vi "discrete_controller.run.vi"(4 "reset? (F)":bool, 5 "error_offset (0)":dbl format="%#_13g", 6 "outut limits (100/0)":cluster{"max_limit":dbl, "min_limit":dbl}={"max_limit"=100.0, "min_limit"=0.0}, 7 "discrete_coefficients":cluster{"b0...bn":dbl[], "a1...an":dbl[]}={"b0...bn"=[0.0, 0.0, 0.0, 0.0], "a1...an"=[0.0, 0.0, 0.0, 0.0]}, 9 "initial_output (0)":dbl format="%#_13g", 10 "feedback":dbl format="%#_13g", 11 "setpoint":dbl format="%#_13g") -> (3 "controller_output":dbl)   [LabVIEW 2015, in "discrete_control_systems.lvlib"]
doc: "This VI implements a SISO discrete controller configured according to the provided discrete coefficients for a difference equation of the form:\n\ny(k) = b0*x(k) + b1*x(k-1) + b2*x(k-2) + bn*x(k-n) - ( a1*y(k-1) + a2*y(k-2) + a3*y(k-3) + an*y(k-n) )\n\nThe output will be coerced withing Min Limit and Max Limit. After resetting the controller, the output will be initialized to the initial output selected. This helps implement bumpless transfers between open loop and closed loop operations."
uses:
  discrete_control_systems.lvlib
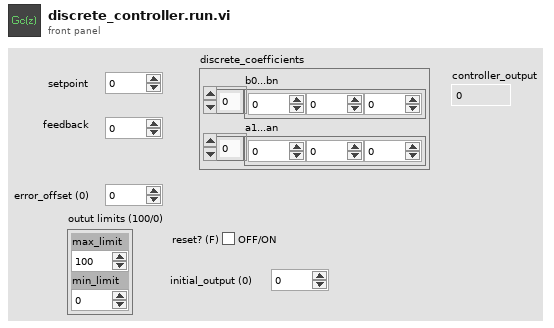
[diagram p1: front panel]
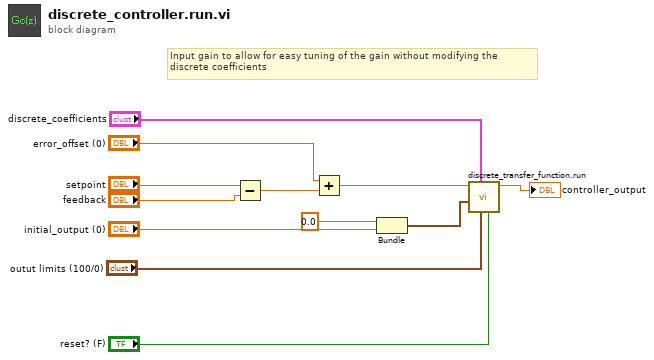
[diagram p0: block diagram]
diagram:
  # "Input gain to allow for easy tuning of the gain without modifying the \ndiscrete coefficients"
  n1 = Subtract(x="setpoint", y="feedback") -> (x-y=w9:dbl)
  n2 = Add(x="error_offset (0)", y=w9) -> (x+y=w4:dbl)
  n3 = Bundle(0.0, "initial_output (0)"="initial_output (0)") -> (w2:cluster{dbl, "initial_output (0)":dbl})  [unwired: 1 in]
  n4 = call "discrete_transfer_function.run.vi"("reset? (F)"="reset? (F)", "outut limits (100/0)"="outut limits (100/0)", "discrete_coefficients"="discrete_coefficients", "initial_values (0)"=w2, "input"=w4) -> ("output"=→"controller_output":dbl)  [unwired: 6 in]
